vi "startUp.vi"(8 "error in (no error)":errorcluster, 10 "HardwareList out":refnum<class "HWConfiguration.lvclass">, 11 "AtomChipHWC in":refnum<class "AtomChipHWC.lvclass">) -> (0 "error out":errorcluster, 3 "AtomChipHWC out":refnum<class "AtomChipHWC.lvclass">)   [LabVIEW 2011, in "Hardware.lvlib" / "HWControllers.lvlib" / "AtomChipHWC.lvclass"]
doc: "Opens the devices ready for use."
uses:
  AtomChipHWC.lvclass
  HardwareConfiguration/HWConfiguration.lvclass
  AtomChipHWC.lvclass/AtomChipHWC.ctl
  Channels/Digital/DigitalOutput.lvclass
  Channels/VoltOutput/AnalogOutput.lvclass
  HWController.lvclass
  Channels/DDSOutput/Generic/DDSOutput.lvclass
  Network Controllers/CameraNetworkController/CameraNetworkController.lvclass
  Network Controllers/NetworkCamera/NetworkCamera.lvclass
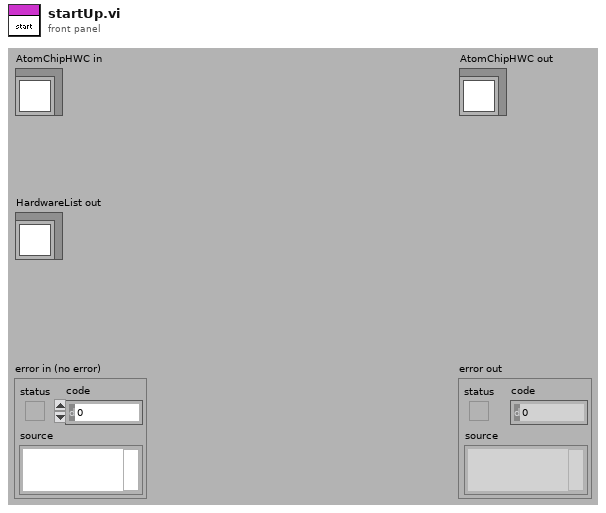
[diagram p1: front panel]
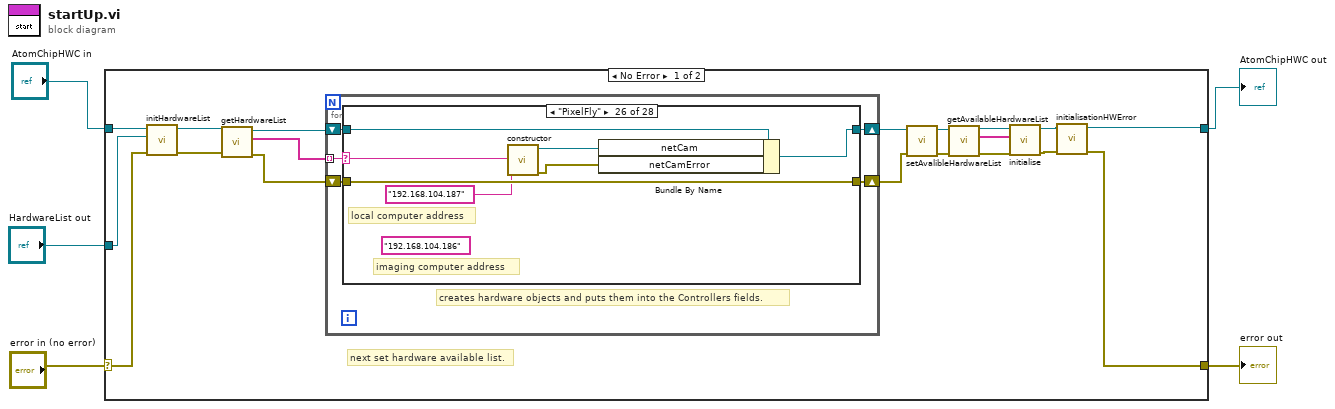
[diagram p0: block diagram]
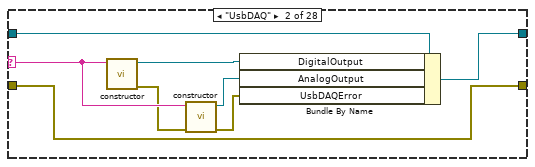
[diagram p3: hidden frame]
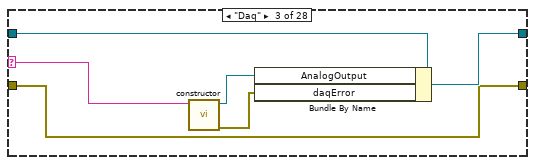
[diagram p4: hidden frame]
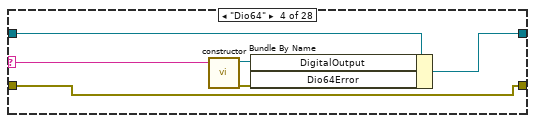
[diagram p5: hidden frame]
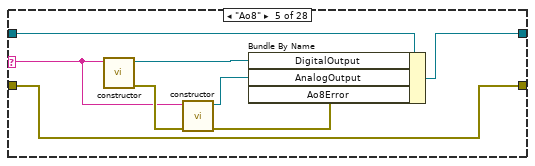
[diagram p6: hidden frame]
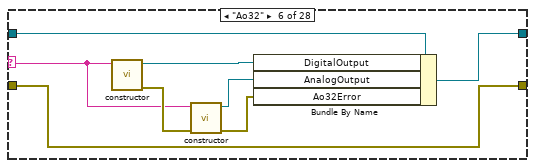
[diagram p7: hidden frame]
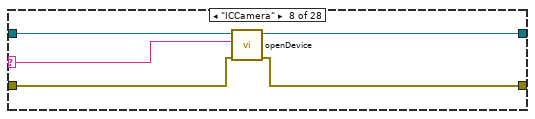
[diagram p9: hidden frame]
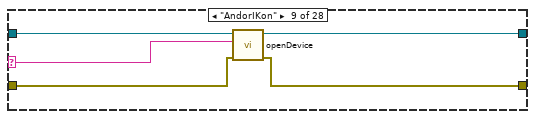
[diagram p10: hidden frame]
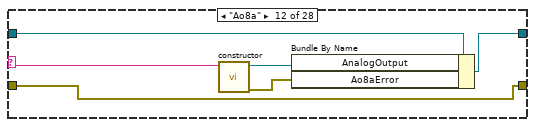
[diagram p13: hidden frame]
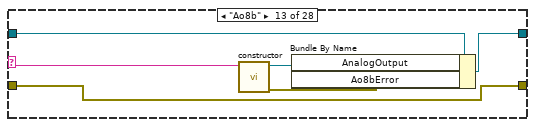
[diagram p14: hidden frame]
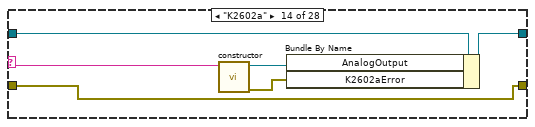
[diagram p15: hidden frame]
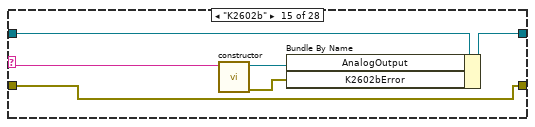
[diagram p16: hidden frame]
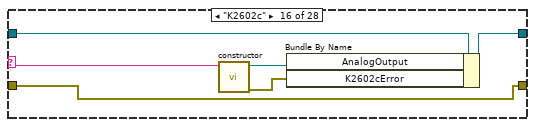
[diagram p17: hidden frame]
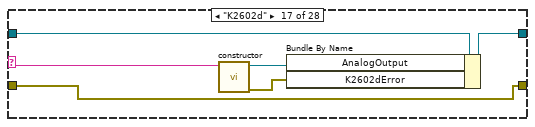
[diagram p18: hidden frame]
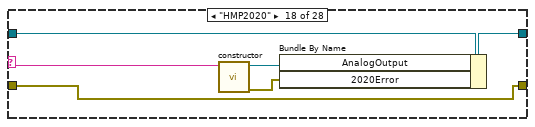
[diagram p19: hidden frame]
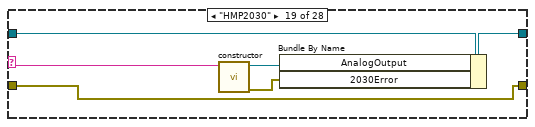
[diagram p20: hidden frame]
diagram:
  n1 = case shown="No Error" "error in (no error)" {
    selector: "error in (no error)" -> [w11 w191]
    tunnel: [w6 w191] -> w4
    tunnel: "AtomChipHWC in" -> [w12 w192]
    tunnel: [w7 w192] -> w2
    tunnel: "HardwareList out" -> [w10 _]
    frame No Error {
      # "next set hardware available list."
      n2 = call-dynamic "initHardwareList.vi"("error in (no error)"=w11, "HardwareList out"=w10, "AtomChipHWC in"=w12) -> ("error out"=w20:errorcluster, "AtomChipHWC out"=w22:refnum<class "AtomChipHWC.lvclass">)  [unwired: 7 in]
      n3 = call "getHardwareList.vi"("error in (no error)"=w20, "HWController.lvclass in"=w22) -> ("error out"=w19:errorcluster, "HardwareList"=w18:string[], "HWController.lvclass out"=w21:refnum<class "AtomChipHWC.lvclass">)  [unwired: 7 in]
      n4 = for {
        tunnel: w18 -> [w25] mode=indexing
        shift-right: [w28] -> w24
        shift-left: w21 -> [w29]
        shift-right: [w26] -> w23
        shift-left: w19 -> [w27]
        # "creates hardware objects and puts them into the Controllers fields."
        n5 = case shown="\"PixelFly\"" w25 {
          selector: w25 -> [_ w39 w42 w48 w56 w62 _ w70 w75 _ _ w86 w92 w98 w104 w110 w116 w123 w128 w134 w140 w146 w152 w158 w164 w171 w178 w190]
          tunnel: w29 -> [w31 w37 w44 w49 w55 w64 w69 w74 w79 w81 w83 w89 w95 w101 w107 w113 w119 w120 w131 w137 w143 w149 w155 w161 w168 w175 w182 w187]
          tunnel: [w31 w34 w43 w50 w54 w63 w69 w73 w78 w81 w83 w88 w94 w100 w106 w112 w118 w125 w130 w136 w142 w148 w154 w160 w167 w174 w181 w186] -> w28
          tunnel: w27 -> [w30 w32 w40 w46 w52 w60 w68 w72 w76 w80 w82 w84 w90 w96 w102 w108 w114 w121 w126 w132 w138 w144 w150 w156 w163 w170 w177 w183]
          tunnel: [w30 w32 w40 w46 w52 w60 w68 w71 w77 w80 w82 w84 w90 w96 w102 w108 w114 w121 w126 w132 w138 w144 w150 w156 w163 w170 w177 w183] -> w26
          frame "No Hardware", Default {
          }
          frame "UsbDAQ" {
            n6 = call "constructor.vi"("deviceName"=w39) -> ("error out"=w38:errorcluster, "DigitalOutput out"=w36:refnum<class "DigitalOutput.lvclass">)  [unwired: 9 in]
            n7 = call "constructor.vi"("error in (no error)"=w38, "deviceName"=w39) -> ("error out"=w33:errorcluster, "AnalogOutput out"=w35:refnum<class "AnalogOutput.lvclass">)  [unwired: 8 in]
            n8 = Bundle By Name(cluster=w37, "DigitalOutput"=w36, "AnalogOutput"=w35, "UsbDAQError"=w33) -> (w34:refnum<class "AtomChipHWC.lvclass">)
          }
          frame "Daq" {
            n9 = call "constructor.vi"("deviceName"=w42) -> ("error out"=w41:errorcluster, "AnalogOutput out"=w45:refnum<class "AnalogOutput.lvclass">)  [unwired: 9 in]
            n10 = Bundle By Name(cluster=w44, "AnalogOutput"=w45, "daqError"=w41) -> (w43:refnum<class "AtomChipHWC.lvclass">)
          }
          frame "Dio64" {
            n11 = call "constructor.vi"("deviceName"=w48) -> ("error out"=w47:errorcluster, "DigitalOutput out"=w51:refnum<class "DigitalOutput.lvclass">)  [unwired: 9 in]
            n12 = Bundle By Name(cluster=w49, "DigitalOutput"=w51, "Dio64Error"=w47) -> (w50:refnum<class "AtomChipHWC.lvclass">)
          }
          frame "Ao8" {
            n13 = call "constructor.vi"("deviceName"=w56) -> ("error out"=w59:errorcluster, "DigitalOutput out"=w58:refnum<class "DigitalOutput.lvclass">)  [unwired: 9 in]
            n14 = call "constructor.vi"("error in (no error)"=w59, "deviceName"=w56) -> ("error out"=w53:errorcluster, "AnalogOutput out"=w57:refnum<class "AnalogOutput.lvclass">)  [unwired: 8 in]
            n15 = Bundle By Name(cluster=w55, "DigitalOutput"=w58, "AnalogOutput"=w57, "Ao8Error"=w53) -> (w54:refnum<class "AtomChipHWC.lvclass">)
          }
          frame "Ao32" {
            n16 = call "constructor.vi"("deviceName"=w62) -> ("error out"=w67:errorcluster, "DigitalOutput out"=w66:refnum<class "DigitalOutput.lvclass">)  [unwired: 9 in]
            n17 = call "constructor.vi"("error in (no error)"=w67, "deviceName"=w62) -> ("error out"=w61:errorcluster, "AnalogOutput out"=w65:refnum<class "AnalogOutput.lvclass">)  [unwired: 8 in]
            n18 = Bundle By Name(cluster=w64, "DigitalOutput"=w66, "AnalogOutput"=w65, "Ao32Error"=w61) -> (w63:refnum<class "AtomChipHWC.lvclass">)
          }
          frame "ArbWave" {
          }
          frame "ICCamera" {
            n19 = call "openDevice.vi"("error in (no error)"=w72, "deviceName"=w70, "AtomChipHWC in"=w74) -> ("error out"=w71:errorcluster, "AtomChipHWC out"=w73:refnum<class "AtomChipHWC.lvclass">)  [unwired: 7 in]
          }
          frame "AndorIKon" {
            n20 = call "openDevice.vi"("error in (no error)"=w76, "deviceName"=w75, "AtomChipHWC in"=w79) -> ("error out"=w77:errorcluster, "AtomChipHWC out"=w78:refnum<class "AtomChipHWC.lvclass">)  [unwired: 7 in]
          }
          frame "S1010" {
          }
          frame "C100" {
          }
          frame "Ao8a" {
            n21 = call "constructor.vi"("deviceName"=w86) -> ("error out"=w85:errorcluster, "AnalogOutput out"=w87:refnum<class "AnalogOutput.lvclass">)  [unwired: 9 in]
            n22 = Bundle By Name(cluster=w89, "AnalogOutput"=w87, "Ao8aError"=w85) -> (w88:refnum<class "AtomChipHWC.lvclass">)
          }
          frame "Ao8b" {
            n23 = call "constructor.vi"("deviceName"=w92) -> ("error out"=w91:errorcluster, "AnalogOutput out"=w93:refnum<class "AnalogOutput.lvclass">)  [unwired: 9 in]
            n24 = Bundle By Name(cluster=w95, "AnalogOutput"=w93, "Ao8bError"=w91) -> (w94:refnum<class "AtomChipHWC.lvclass">)
          }
          frame "K2602a" {
            n25 = call "constructor.vi"("deviceName"=w98) -> ("error out"=w97:errorcluster, "AnalogOutput out"=w99:refnum<class "AnalogOutput.lvclass">)  [unwired: 9 in]
            n26 = Bundle By Name(cluster=w101, "AnalogOutput"=w99, "K2602aError"=w97) -> (w100:refnum<class "AtomChipHWC.lvclass">)
          }
          frame "K2602b" {
            n27 = call "constructor.vi"("deviceName"=w104) -> ("error out"=w103:errorcluster, "AnalogOutput out"=w105:refnum<class "AnalogOutput.lvclass">)  [unwired: 9 in]
            n28 = Bundle By Name(cluster=w107, "AnalogOutput"=w105, "K2602bError"=w103) -> (w106:refnum<class "AtomChipHWC.lvclass">)
          }
          frame "K2602c" {
            n29 = call "constructor.vi"("deviceName"=w110) -> ("error out"=w109:errorcluster, "AnalogOutput out"=w111:refnum<class "AnalogOutput.lvclass">)  [unwired: 9 in]
            n30 = Bundle By Name(cluster=w113, "AnalogOutput"=w111, "K2602cError"=w109) -> (w112:refnum<class "AtomChipHWC.lvclass">)
          }
          frame "K2602d" {
            n31 = call "constructor.vi"("deviceName"=w116) -> ("error out"=w115:errorcluster, "AnalogOutput out"=w117:refnum<class "AnalogOutput.lvclass">)  [unwired: 9 in]
            n32 = Bundle By Name(cluster=w119, "AnalogOutput"=w117, "K2602dError"=w115) -> (w118:refnum<class "AtomChipHWC.lvclass">)
          }
          frame "HMP2020" {
            n33 = call "constructor.vi"("deviceName"=w123) -> ("error out"=w122:errorcluster, "AnalogOutput out"=w124:refnum<class "AnalogOutput.lvclass">)  [unwired: 9 in]
            n34 = Bundle By Name(cluster=w120, "AnalogOutput"=w124, "2020Error"=w122) -> (w125:refnum<class "AtomChipHWC.lvclass">)
          }
          frame "HMP2030" {
            n35 = call "constructor.vi"("deviceName"=w128) -> ("error out"=w127:errorcluster, "AnalogOutput out"=w129:refnum<class "AnalogOutput.lvclass">)  [unwired: 9 in]
            n36 = Bundle By Name(cluster=w131, "AnalogOutput"=w129, "2030Error"=w127) -> (w130:refnum<class "AtomChipHWC.lvclass">)
          }
          frame "HMP4030" {
            n37 = call "constructor.vi"("deviceName"=w134) -> ("error out"=w133:errorcluster, "AnalogOutput out"=w135:refnum<class "AnalogOutput.lvclass">)  [unwired: 9 in]
            n38 = Bundle By Name(cluster=w137, "AnalogOutput"=w135, "4030Error"=w133) -> (w136:refnum<class "AtomChipHWC.lvclass">)
          }
          frame "SpinCoreDDS0" {
            n39 = call "constructor.vi"("device"=w140) -> ("error out"=w139:errorcluster, "DDSOutput out"=w141:refnum<class "DDSOutput.lvclass">)  [unwired: 9 in]
            n40 = Bundle By Name(cluster=w143, "DDSOutput"=w141, "DDS0Error"=w139) -> (w142:refnum<class "AtomChipHWC.lvclass">)
          }
          frame "SpinCoreDDS1" {
            n41 = call "constructor.vi"("device"=w146) -> ("error out"=w145:errorcluster, "DDSOutput out"=w147:refnum<class "DDSOutput.lvclass">)  [unwired: 9 in]
            n42 = Bundle By Name(cluster=w149, "DDSOutput"=w147, "DDS1Error"=w145) -> (w148:refnum<class "AtomChipHWC.lvclass">)
          }
          frame "k3390" {
            n43 = call "constructor.vi"("device"=w152) -> ("error out"=w151:errorcluster, "DDSOutput out"=w153:refnum<class "DDSOutput.lvclass">)  [unwired: 9 in]
            n44 = Bundle By Name(cluster=w155, "DDSOutput"=w153, "DDS1Error"=w151) -> (w154:refnum<class "AtomChipHWC.lvclass">)
          }
          frame "CQTDDS0" {
            n45 = call "constructor.vi"("device"=w158) -> ("error out"=w157:errorcluster, "DDSOutput out"=w159:refnum<class "DDSOutput.lvclass">)  [unwired: 9 in]
            n46 = Bundle By Name(cluster=w161, "DDSOutput"=w159, "DDS0Error"=w157) -> (w160:refnum<class "AtomChipHWC.lvclass">)
          }
          frame "Pixis" {
            (unwired) "192.168.104.186" ("remote address")
            # "local computer address"
            # "imaging computer address"
            n47 = call "constructor.vi"("machine name"="192.168.104.187" ("remote address"), "Camera"=w164) -> ("error out"=w165:errorcluster, "NetworkCamera out"=w166:refnum<class "NetworkCamera.lvclass">)  [unwired: 8 in]
            n48 = Bundle By Name(cluster=w168, "netCam"=w166, "netCamError"=w165) -> (w167:refnum<class "AtomChipHWC.lvclass">)
          }
          frame "PixelFly" {
            (unwired) "192.168.104.186" ("remote address")
            # "local computer address"
            # "imaging computer address"
            n49 = call "constructor.vi"("machine name"="192.168.104.187" ("remote address"), "Camera"=w171) -> ("error out"=w172:errorcluster, "NetworkCamera out"=w173:refnum<class "NetworkCamera.lvclass">)  [unwired: 8 in]
            n50 = Bundle By Name(cluster=w175, "netCam"=w173, "netCamError"=w172) -> (w174:refnum<class "AtomChipHWC.lvclass">)
          }
          frame "ProEM" {
            (unwired) "192.168.104.171" ("remote address")
            # "imaging computer address"
            # "my laptop address"
            n51 = call "constructor.vi"("machine name"="192.168.104.186" ("remote address"), "Camera"=w178) -> ("error out"=w179:errorcluster, "NetworkCamera out"=w180:refnum<class "NetworkCamera.lvclass">)  [unwired: 8 in]
            n52 = Bundle By Name(cluster=w182, "netCam"=w180, "netCamError"=w179) -> (w181:refnum<class "AtomChipHWC.lvclass">)
          }
          frame "oldPixelfly", "oldProEM_WinX32" {
            n53 = call "constructor.vi"("remote port"=u16 6340, "remote address"="192.168.104.186", "camera"=w190) -> ("error out"=w184:errorcluster, "CameraNetworkController out"=w185:refnum<class "CameraNetworkController.lvclass">)  [unwired: 7 in]
            n54 = Bundle By Name(cluster=w187, "CameraNetworkController"=w185, "CameraNError"=w184) -> (w186:refnum<class "AtomChipHWC.lvclass">)
          }
        }
      }
      n55 = call "setAvalibleHardwareList.vi"("error in (no error)"=w23, "HWController in"=w24) -> ("error out"=w16:errorcluster, "HWController out"=w17:refnum<class "AtomChipHWC.lvclass">)  [unwired: 8 in]
      n56 = call "getAvailableHardwareList.vi"("error in (no error)"=w16, "HWController.lvclass in"=w17) -> ("error out"=w14:errorcluster, "AvailableHardwareList"=w13:string[], "HWController.lvclass out"=w15:refnum<class "AtomChipHWC.lvclass">)  [unwired: 7 in]
      n57 = call-dynamic "initialise.vi"("error in (no error)"=w14, "HWList"=w13, "AtomChipHWC in"=w15) -> ("error out"=w8:errorcluster, "AtomChipHWC out"=w9:refnum<class "AtomChipHWC.lvclass">)  [unwired: 7 in]
      n58 = call-dynamic "initialisationHWError.vi"("error in (no error)"=w8, "AtomChipHWC in"=w9) -> ("error out"=w6:errorcluster, "AtomChipHWC out"=w7:refnum<class "AtomChipHWC.lvclass">)  [unwired: 8 in]
    }
    frame Error {
    }
  }
  "error out" <- w4
  "AtomChipHWC out" <- w2
